vi "axex_is_workbook_opened.vi"(8 "error in":errorcluster, 11 "path":path) -> (0 "error out":errorcluster, 3 "is loaded?":bool)   [LabVIEW 2020, in "AX Excel.lvlib"]
doc: "Returns true if given file is loaded in M$ Excel."
uses:
  AX Excel.lvlib
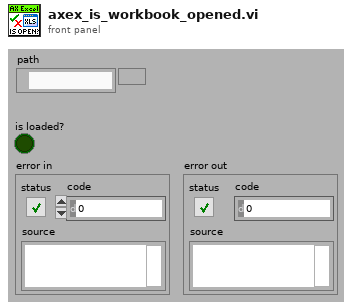
[diagram p1: front panel]
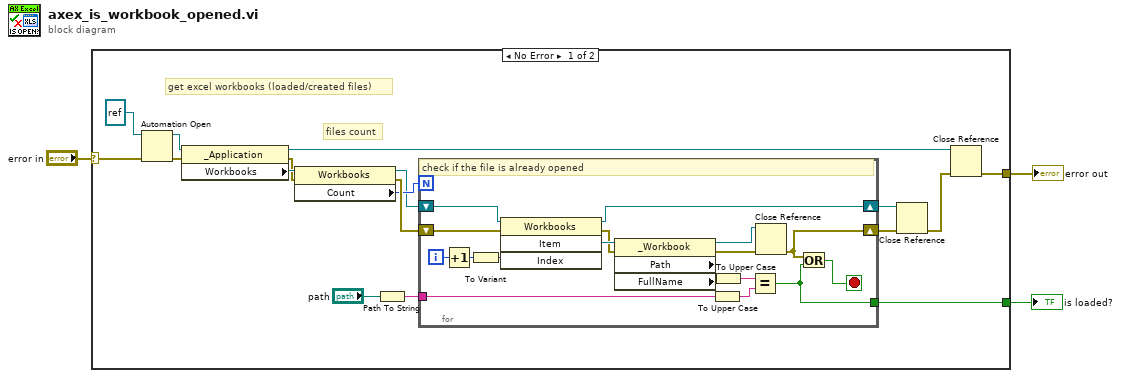
[diagram p0: block diagram]
diagram:
  n1 = case shown="No Error" "error in" {
    selector: "error in" -> [w4 w38]
    tunnel: [w10 w38] -> w3
    tunnel: [w6 _] -> w2
    frame No Error {
      # "files count"
      # "get excel workbooks (loaded/created files)"
      n2 = Automation Open(error in (no error)=w4, Automation Refnum=refnum<k7> refnum ("Excel._Application")) -> (Automation Refnum=w18:refnum<k7>, error out=w19:errorcluster)  [unwired: 2 in]
      n3 = property class="_Application"(reference=w18, error in=w19) -> (reference out=w17:refnum<k7>, error out=w12:errorcluster, "Workbooks"=w14:refnum<k7>)
      n4 = property class="Workbooks"(reference=w14, error in=w12) -> (reference out=w9:refnum<k7>, error out=w16:errorcluster, "Count"=w15:i32)
      n5 = Path To String(path="path") -> (string=w13:string)
      n6 = for {
        N: w15 -> [_]
        shift-right: [w23] -> w8
        shift-left: w16 -> [w36]
        tunnel: w13 -> [w27]
        tunnel: [w24] -> w6
        shift-right: [w26] -> w7
        shift-left: w9 -> [w34]
        i -> [w32]
        stop <- w25 stop-if-true
        # "check if the file is already opened"
        n7 = Increment(x=w32) -> (x+1=w31:i32)
        n8 = To Variant(anything=w31) -> (Variant=w33:variant)
        n9 = invoke class="Workbooks" method="Item"(reference=w34, error in=w36, "Index"=w33) -> (reference out=w26:refnum<k7>, error out=w35:errorcluster, "Item"=w37:refnum<k7>)  [unwired: 1 in, 1 out]
        n10 = property class="_Workbook" props=["Path", "FullName"](reference=w37, error in=w35) -> (reference out=w29:refnum<k7>, error out=w30:errorcluster, "FullName"=w28:string)  [unwired: 1 out]
        n11 = To Upper Case(1:w27) -> (0:w21:string)
        n12 = To Upper Case(1:w28) -> (0:w22:string)
        n13 = Equal?(x=w22, y=w21) -> (x = y?=w24:bool)
        n14 = Close Reference(reference=w29, error in (no error)=w30) -> (error out=w23:errorcluster)
        n15 = Or(x=w23, y=w24) -> (x .or. y?=w25:bool)
      }
      n16 = Close Reference(reference=w7, error in (no error)=w8) -> (error out=w11:errorcluster)
      n17 = Close Reference(reference=w17, error in (no error)=w11) -> (error out=w10:errorcluster)
    }
    frame Error {
    }
  }
  "error out" <- w3
  "is loaded?" <- w2
